vi "Factory Build Up.vi"(8 "error in (no error)":errorcluster, 9 "Factory Set In":T1, 10 "System Module Factory In":refnum<class "System Modules Factory.lvclass">, 11 "Node Actor in":refnum<class "Node Actor.lvclass">) -> (0 "error out":errorcluster, 2 "System Module Factory Out":refnum<class "System Modules Factory.lvclass">, 3 "Node Actor out":refnum<class "Node Actor.lvclass">)   [LabVIEW 2024, in "Node Actor.lvclass"]
uses:
  Node Actor.lvclass
  Factory/System Modules Factory/System Modules Factory.lvclass
  Factory/Node Controller Factory/Node Controller Factory.lvclass
  Actor Assistant/Notifier/Notifier.lvclass
  Factory/Messenger Factory/Messenger Factory.lvclass
  Node Actor.lvclass/Node Actor.ctl
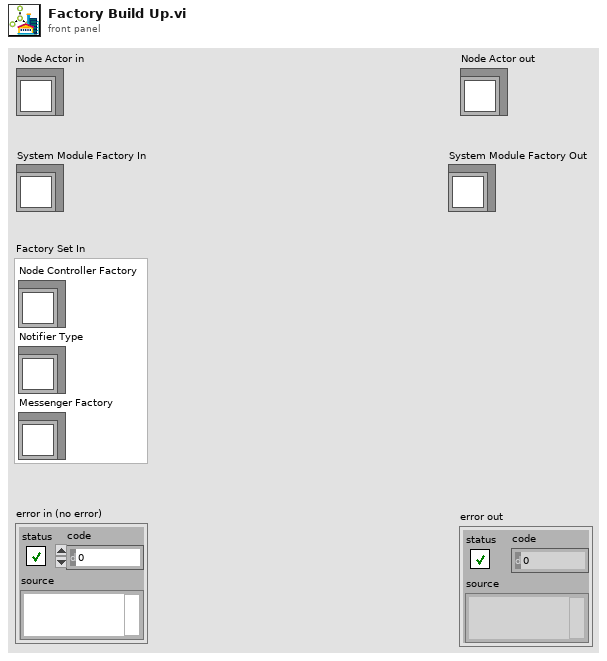
[diagram p1: front panel]
types:
  T1 = cluster{"Node Controller Factory":refnum<class "Node Controller Factory.lvclass">, "Notifier Type":refnum<class "Notifier.lvclass">, "Messenger Factory":refnum<class "Messenger Factory.lvclass">}
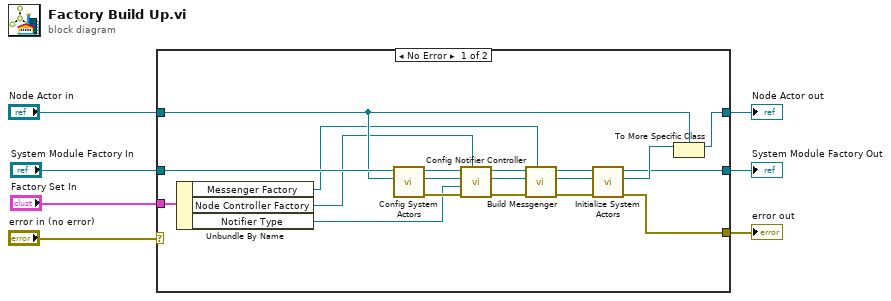
[diagram p0: block diagram]
diagram:
  n1 = case shown="No Error" "error in (no error)" {
    selector: "error in (no error)" -> [_ w29]
    tunnel: [w16 w29] -> w6
    tunnel: [w12 w28] -> w4
    tunnel: "Node Actor in" -> [w13 w28]
    tunnel: "System Module Factory In" -> [w23 w27]
    tunnel: [w14 w27] -> w2
    tunnel: "Factory Set In" -> [w11 _]
    frame No Error {
      n2 = Unbundle By Name(w11) -> ("Messenger Factory"=w9:refnum<class "Messenger Factory.lvclass">, "Node Controller Factory"=w10:refnum<class "Node Controller Factory.lvclass">, "Notifier Type"=w8:refnum<class "Notifier.lvclass">)
      n3 = call-dynamic "Config System Actors.vi"("Root Actor In"=w13, "System Modules Factory in"=w23) -> ("error out"=w25:errorcluster, "Root Actor Out"=w17:refnum<class "Root Actor.lvclass">, "System Modules Factory out"=w22:refnum<class "System Modules Factory.lvclass">)  [unwired: 7 in]
      n4 = call-dynamic "Config Notifier Controller.vi"("Node Controller Factory In"=w10, "error in (no error)"=w25, "Notifier Type"=w8, "Root Actor In"=w17, "System Modules Factory in"=w22) -> ("error out"=w26:errorcluster, "Root Actor Out"=w18:refnum<class "Root Actor.lvclass">, "System Modules Factory out"=w21:refnum<class "System Modules Factory.lvclass">)  [unwired: 3 in, 1 out]
      n5 = call-dynamic "Build Messgenger.vi"("Messenger Factory in"=w9, "error in (no error)"=w26, "Root Actor In"=w18, "System Modules Factory In"=w21) -> ("error out"=w24:errorcluster, "Root Actor Out"=w19:refnum<class "Root Actor.lvclass">, "System Modules Factory Out"=w20:refnum<class "System Modules Factory.lvclass">)  [unwired: 4 in, 1 out]
      n6 = call-dynamic "Initialize System Actors.vi"("error in (no error)"=w24, "Root Actor In"=w19, "System Modules Factory in"=w20) -> ("error out"=w16:errorcluster, "Root Actor Out"=w15:refnum<class "Root Actor.lvclass">, "System Modules Factory out"=w14:refnum<class "System Modules Factory.lvclass">)  [unwired: 6 in]
      n7 = To More Specific Class(target class=w13, reference=w15) -> (specific class reference=w12:refnum<class "Node Actor.lvclass">)  [unwired: 1 in, 1 out]
    }
    frame Error {
    }
  }
  "error out" <- w6
  "Node Actor out" <- w4
  "System Module Factory Out" <- w2
